vi "Read datatype.vi"(8 "error in (no error)":errorcluster, 11 "JSON Array in":refnum<class "JSON Array.lvclass">) -> (0 "error out":errorcluster, 2 "datatype":T1, 3 "JSON Array out":refnum<class "JSON Array.lvclass">)   [LabVIEW 2017, in "LVJSON.lvlib" / "JSON Array.lvclass"]
uses:
  JSON Array.lvclass
  JSON Types.ctl
  LVJSON.lvlib
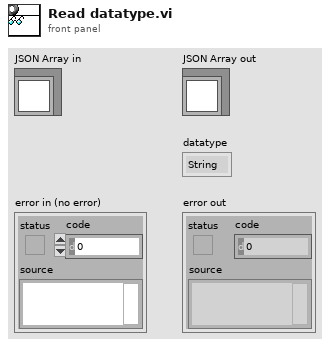
[diagram p1: front panel]
types:
  T1 = typedef "LVJSON.lvlib/JSON Types.ctl" = enum16{"String", "Numeric", "Boolean", "NULL", "Object", "1D Array", "Unknown"}
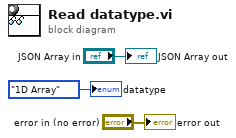
[diagram p0: block diagram]
diagram:
  "error out" <- "error in (no error)"
  "JSON Array out" <- "JSON Array in"
  "datatype" <- JSON_Types."1D Array" ("datatype")
